vi "PPS Init.vi"(8 "error in (no error)":errorcluster, 10 "VISA resource name":refnum<visa-resource-name>, 11 "PowerSupply in":refnum<class "PowerSupply.lvclass">) -> (0 "error out":errorcluster, 3 "PowerSupply out":refnum<class "PowerSupply.lvclass">)   [LabVIEW 2023, in "HardwareAbstractionLayer_LVOOP.lvlib" / "PowerSupply.lvclass"]
uses:
  PowerSupply.lvclass
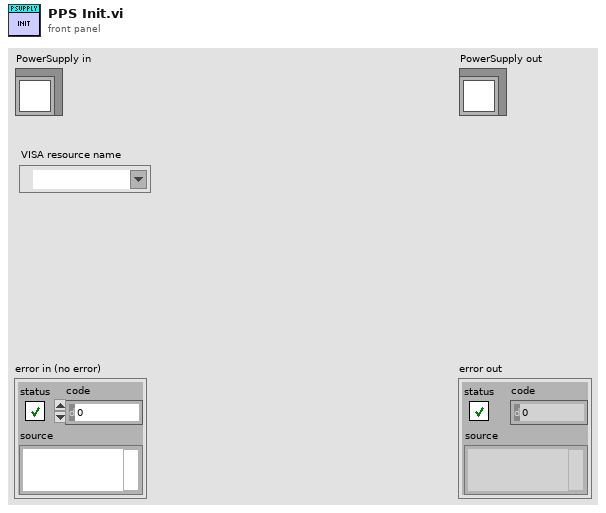
[diagram p1: front panel]
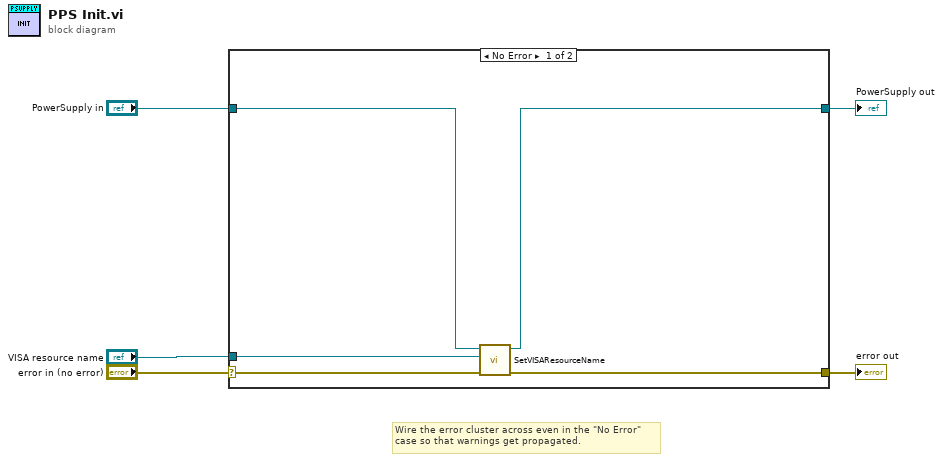
[diagram p0: block diagram]
diagram:
  # "Wire the error cluster across even in the \"No Error\"\ncase so that warnings get propagated."
  n1 = case shown="No Error" "error in (no error)" {
    selector: "error in (no error)" -> [w10 w12]
    tunnel: [w7 w12] -> w4
    tunnel: [w8 w11] -> w2
    tunnel: "PowerSupply in" -> [w9 w11]
    tunnel: "VISA resource name" -> [w6 _]
    frame No Error {
      n2 = call-dynamic "SetVISAResourceName.vi"("error in (no error)"=w10, "VISA resource name"=w6, "object in"=w9) -> ("error out"=w7:errorcluster, "object out"=w8:refnum<class "PowerSupply.lvclass">)  [unwired: 7 in]
    }
    frame Error {
    }
  }
  "error out" <- w4
  "PowerSupply out" <- w2
